vi "Half adder.vi"(10 "Input in":bool, 11 "Input 1":bool) -> (2 "Boolean":bool, 3 "Boolean 2":bool)   [LabVIEW 2018]
doc: "This SUB VI takes two input as gives the sum as well as carry of the two bollean values"
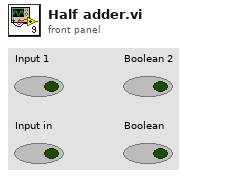
[diagram p1: front panel]
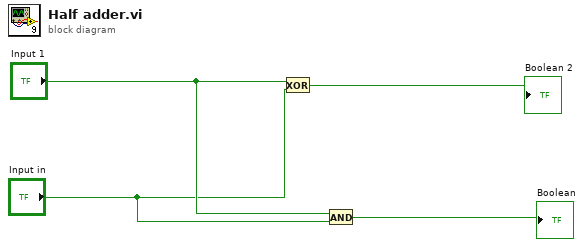
[diagram p0: block diagram]
diagram:
  n1 = Exclusive Or(1:"Input in", 2:"Input 1") -> (0:→"Boolean 2":bool)
  n2 = And(x="Input 1", y="Input in") -> (x .and. y?=→"Boolean":bool)
